vi "Shutdown.vi"(8 "error in":errorcluster, 11 "Instrument in":refnum<class "Instrument.lvclass">) -> (0 "error out":errorcluster, 3 "Instrument out":refnum<class "Instrument.lvclass">)   [LabVIEW 2019, in "Instrument.lvclass"]
doc: "General Instrument shutdown procedures. Kill open queues."
uses:
  Instrument.lvclass
  Session Log/System Log.lvclass
  C:/Program Files (x86)/National Instruments/LabVIEW 2019/vi.lib/MSR Consulting, LLC/General Reuse/Session APIs/_Session Fwk/Session - Root.lvclass
  Session APIs/File Access/Config Data/Config Data.lvclass
  Instrument.lvclass/Instrument.ctl
  <vilib>/MSR Consulting, LLC/General Reuse/Session APIs/_Session Fwk/Session - Root.lvclass
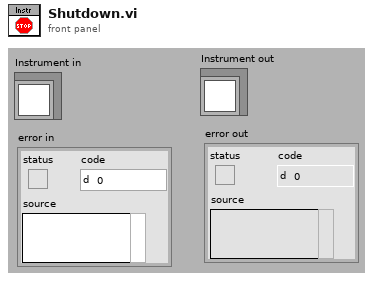
[diagram p1: front panel]
types:
  T1 = typedef "Session - Root.lvclass/Session Handle.ctl" = refnum<data-value>
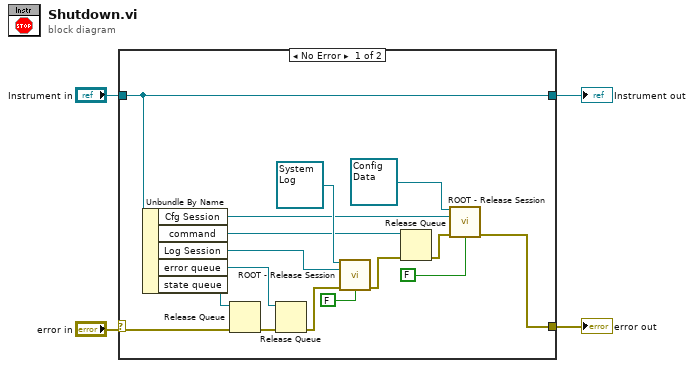
[diagram p0: block diagram]
diagram:
  n1 = case shown="No Error" "error in" {
    selector: "error in" -> [w18 w22]
    tunnel: [w5 w22] -> w3
    tunnel: [w20 w21] -> w1
    tunnel: "Instrument in" -> [w20 w21]
    frame No Error {
      n2 = Unbundle By Name(w20) -> ("Cfg Session"=w9:T1, "command"=w11:refnum<queue>, "Log Session"=w15:T1, "error queue"=w17:refnum<queue>, "state queue"=w19:refnum<queue>)
      n3 = Release Queue(queue=w19, error in (no error)=w18) -> (error out=w16:errorcluster)  [unwired: 1 in, 2 out]
      n4 = Release Queue(queue=w17, error in (no error)=w16) -> (error out=w14:errorcluster)  [unwired: 1 in, 2 out]
      n5 = call <vilib>:"ROOT - Release Session.vi"("OBJ - Session in"=refnum<class "System Log.lvclass"> refnum ("Sys Log"), "Session Handle in"=w15, "error in (no error)"=w14, "force destroy? (F)"=FALSE) -> ("error out"=w10:errorcluster)  [unwired: 10 in, 1 out]
      n6 = Release Queue(queue=w11, error in (no error)=w10) -> (error out=w6:errorcluster)  [unwired: 1 in, 2 out]
      n7 = call <vilib>:"ROOT - Release Session.vi"("OBJ - Session in"=refnum<class "Config Data.lvclass"> refnum ("Config Data"), "Session Handle in"=w9, "error in (no error)"=w6, "force destroy? (F)"=FALSE) -> ("error out"=w5:errorcluster)  [unwired: 10 in, 1 out]
    }
    frame Error {
    }
  }
  "error out" <- w3
  "Instrument out" <- w1
